vi "mask.vi"(10 "mask":u8[](array[numeric]), 11 "data in":string) -> (3 "masked data":string)   [LabVIEW 2019, in "WebSocket Server Toolkit.lvlib"]
uses:
  WebSocket Server Toolkit.lvlib
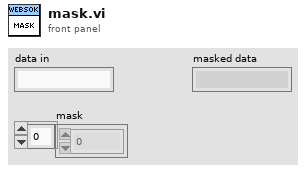
[diagram p1: front panel]
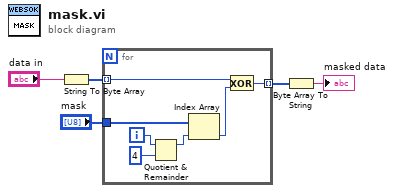
[diagram p0: block diagram]
diagram:
  n1 = String To Byte Array(string="data in") -> (unsigned byte array=w3:u8[])
  n2 = for {
    tunnel: w3 -> [w8] mode=indexing
    tunnel: "mask" -> [w12]
    tunnel: [w6] -> w5 mode=indexing
    i -> [w11]
    n3 = Quotient & Remainder(x=w11, y=4) -> (x-y*floor(x/y)=w9:i32)  [unwired: 1 out]
    n4 = Index Array(array=w12, index=w9) -> (element=w7:u8)
    n5 = Exclusive Or(1:w7, 2:w8) -> (0:w6:u8)
  }
  n6 = Byte Array To String(unsigned byte array=w5) -> (string=→"masked data":string)
